vi "run.vi"() -> ()   [LabVIEW 2010, in "AnalysisRaps2.lvclass"]
uses:
  AnalysisRaps2.lvclass
  common/classes/ErrorController/ErrorController/ErrorController.lvclass
  common/classes/ImageCollection/ImageCollection/ImageCollection.lvclass
  AnalysisRaps2.lvclass/AnalysisRaps2.ctl
  common/classes/ErrorController/ErrorController/class_data.vi
panel:
  out "average":sgl[](graph) caption="graph r"
  in  "stop":bool
  out "graph r":sgl[][](graph)
  out "r0":sgl[](array[numeric])
  in  "r0 end point":i32=1
  in  "r0 start point":i32
  in  "# rolling average":i32=1 min=1
  in  "extra offset":dbl=10.0
  in  "show index":i32
  out "single graph":sgl[](graph)
  out "graph blue":sgl[][](graph)
  in  "# lines to skip":i32
  out "graph yellow":sgl[][](graph)
  in  "# subpatterns":i32=1 min=1
  out "progress slider":u8(slide) scale=0.0..100.0
  in  "channel: yellow":i32=1
  in  "channel: blue":i32
  out "error out":errorcluster
  in  "Path":path
  out "error handler":bool
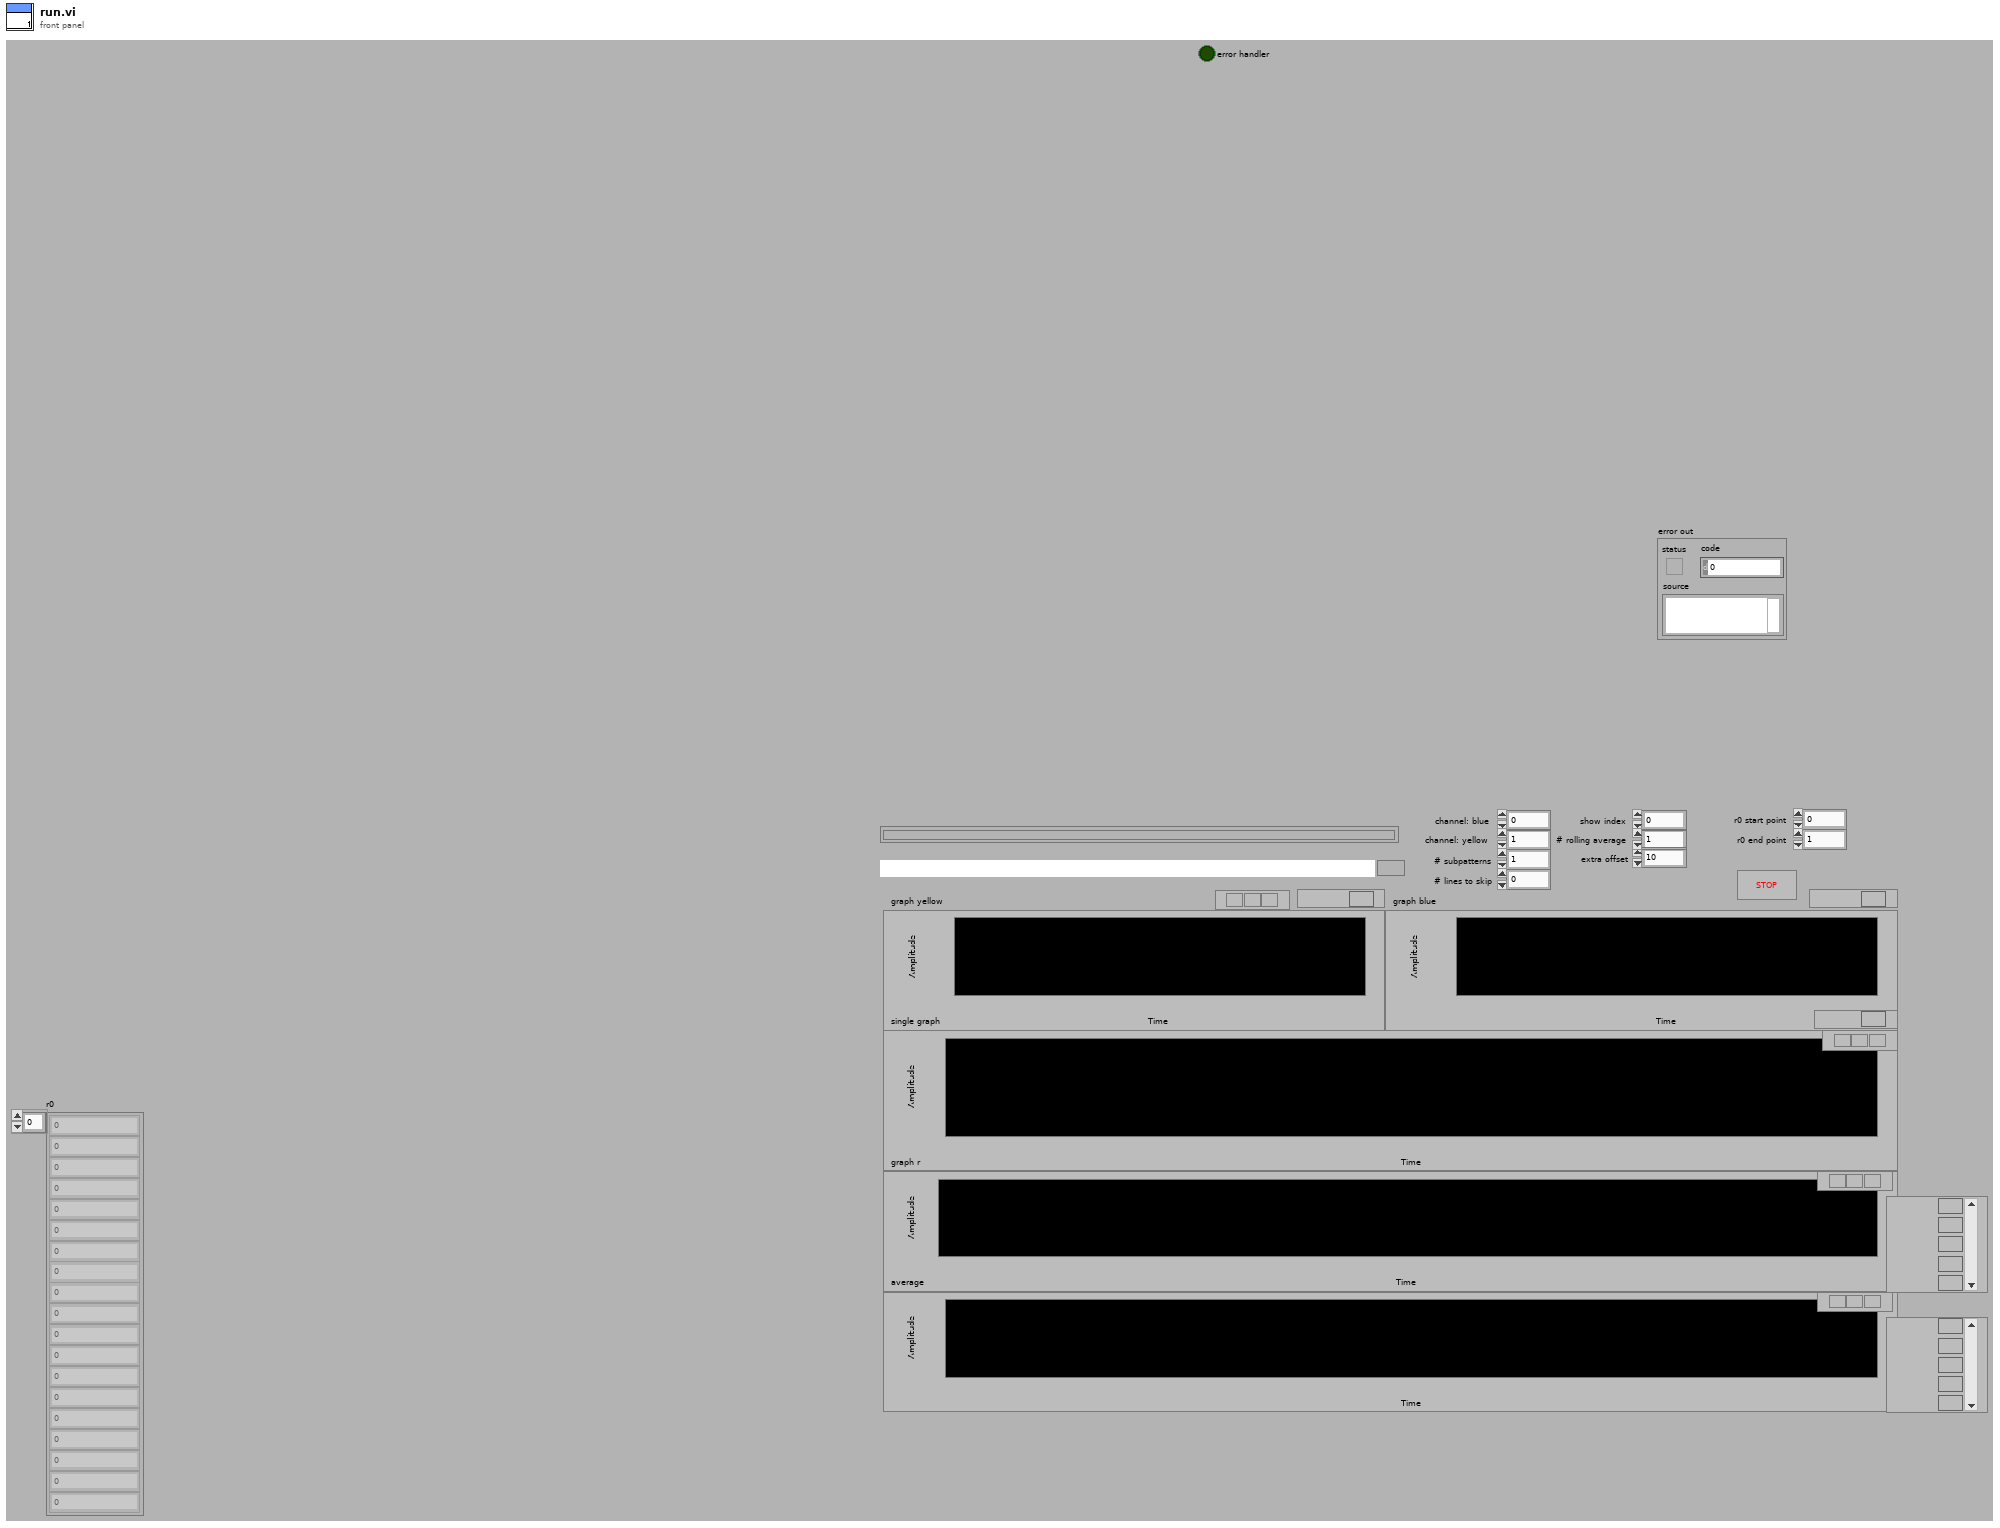
[diagram p1: front panel]
types:
  T1 = typedef "Image Type" = u32
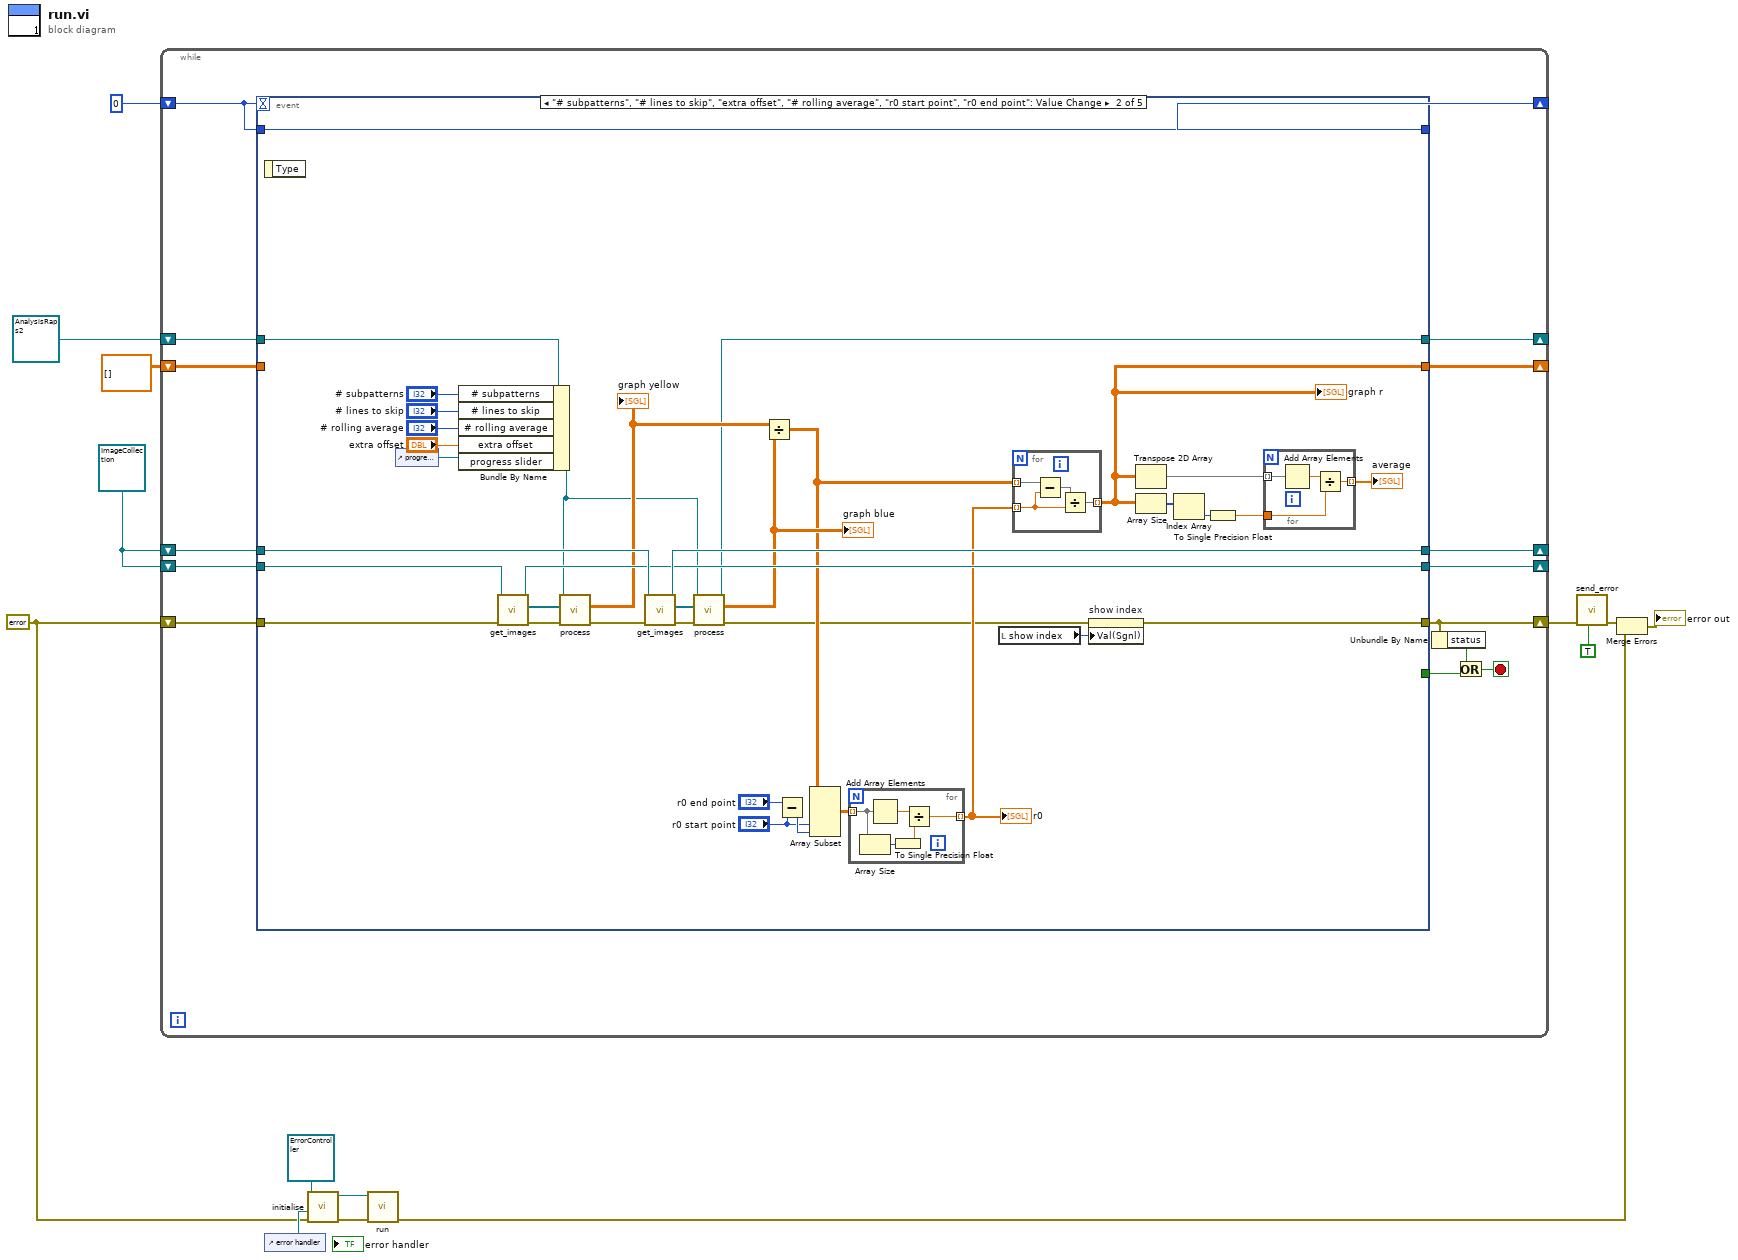
[diagram p0: block diagram]
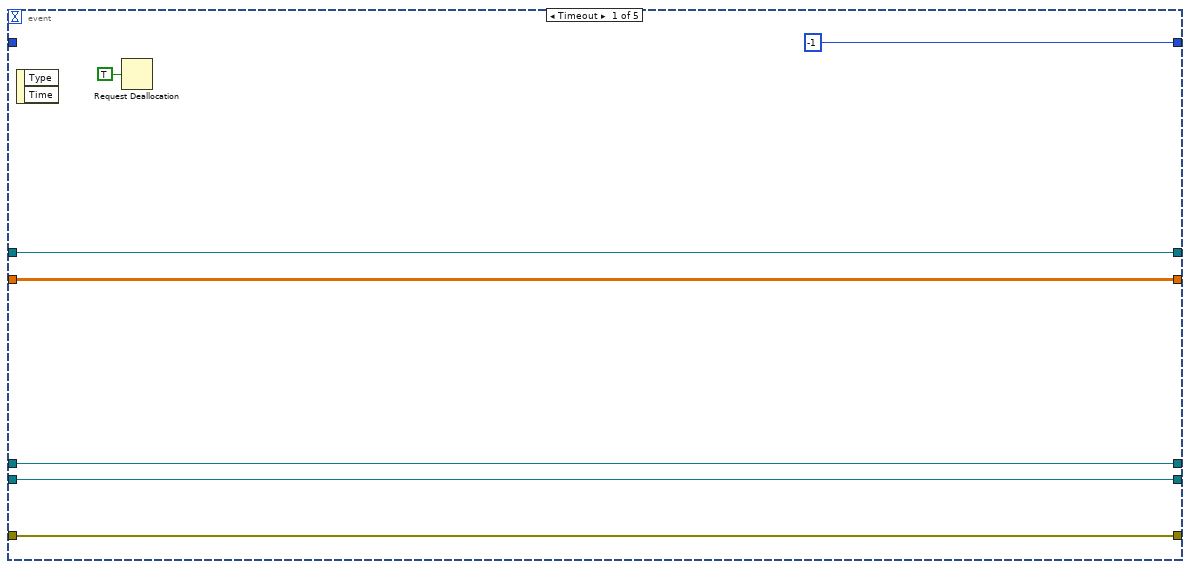
[diagram p2: hidden frame]
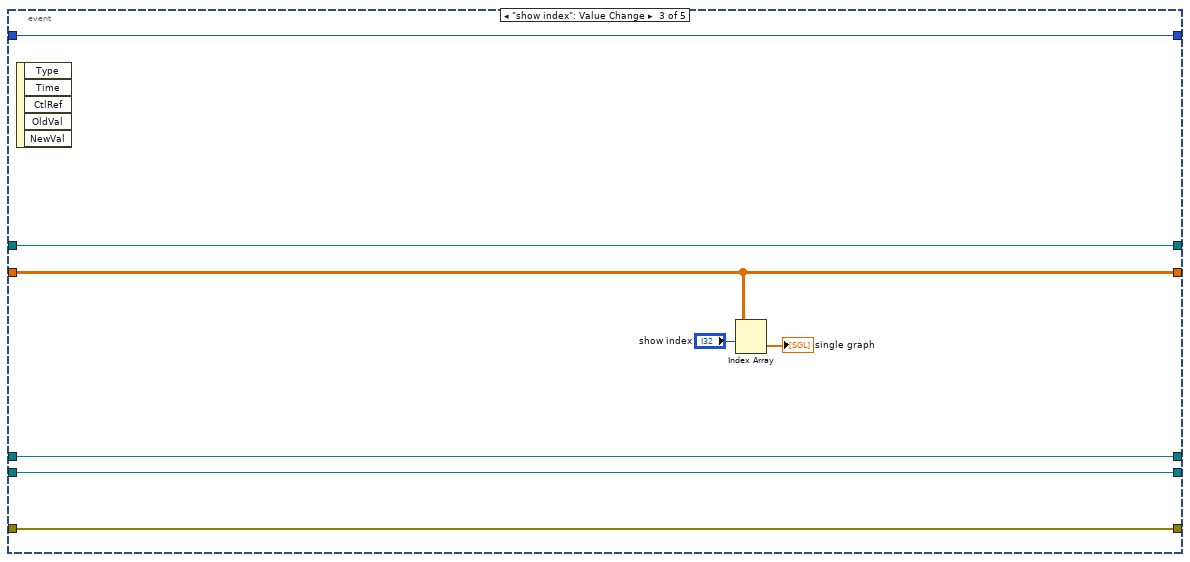
[diagram p3: hidden frame]
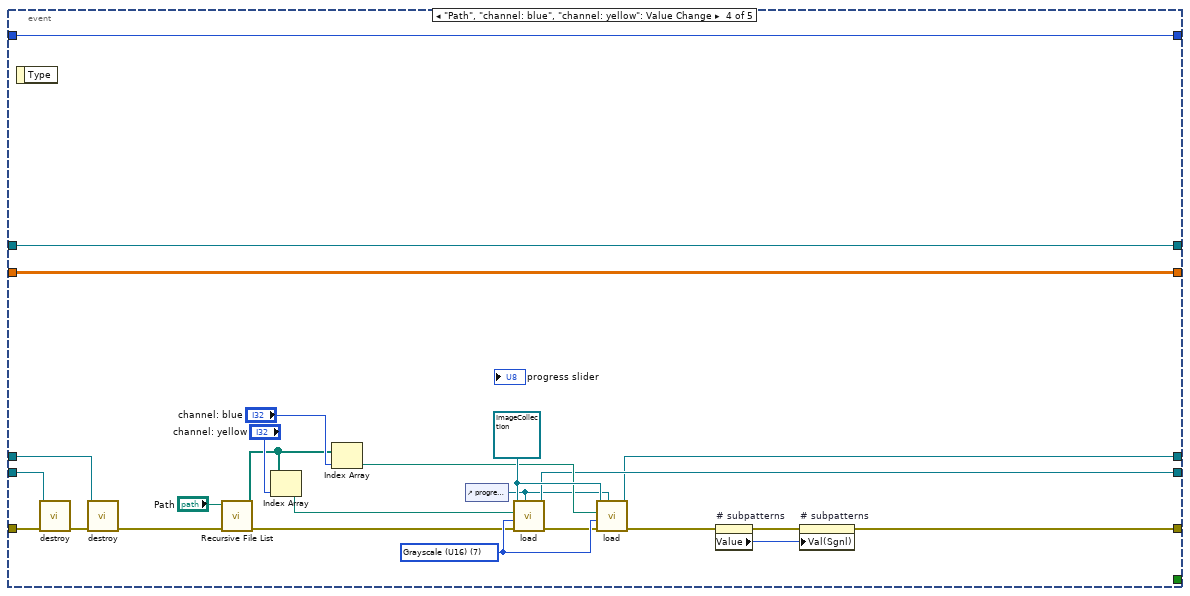
[diagram p4: hidden frame]
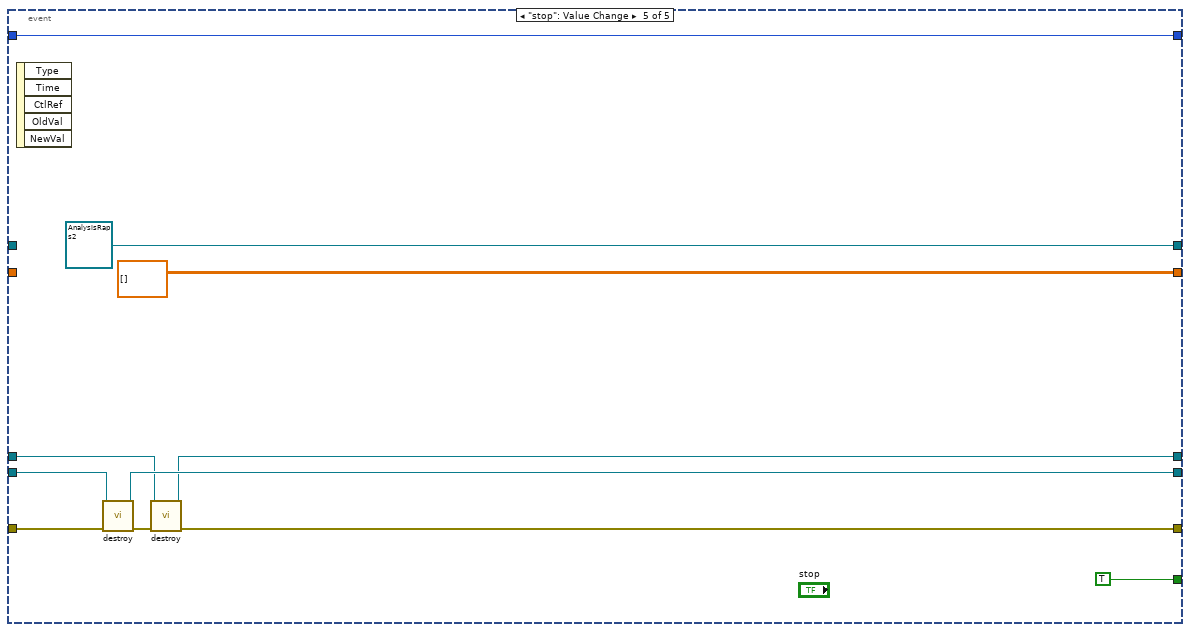
[diagram p5: hidden frame]
diagram:
  w1 = refnum<class "ImageCollection.lvclass"> refnum ("ImageCollection out")
  w9 = errorcluster {"status"=FALSE, "code"=0, "source"=""} ("error in (no error)")
  n1 = while {
    shift-right: [w29] -> _
    shift-left: 0 -> [w28]
    shift-right: [w18] -> w7
    shift-left: w9 -> [w27]
    shift-right: [w25] -> _
    shift-left: refnum<class "AnalysisRaps2.lvclass"> refnum ("AnalysisRaps2.lvclass") -> [w26]
    shift-right: [w22] -> _
    shift-left: w1 -> [w23]
    shift-right: [w21] -> _
    shift-left: w1 -> [w24]
    shift-right: [w20] -> _
    shift-left: sgl[][] [] -> [w19]
    stop <- w15 stop-if-true
    n2 = event shown="[1] \"# subpatterns\", \"# lines to skip\", \"extra offset\", \"# rolling average\", \"r0 start point\", \"r0 end point\": Value Change" {
      selector: _ -> [_ _ _ _ _]
      dyn-events: _ -> [_ _ _ _ _]
      timeout: w28 -> [_ _ _ _ _]
      tunnel: [-1 w72 w93 w118 w129] -> w29
      tunnel: w28 -> [_ w72 w93 w118 w129]
      tunnel: w27 -> [w34 w47 w92 w103 w126]
      tunnel: [w34 w49 w92 w97 w125] -> w18
      tunnel: w26 -> [w33 w60 w91 w117 _]
      tunnel: [w33 w61 w91 w117 refnum<class "AnalysisRaps2.lvclass"> refnum ("AnalysisRaps2.lvclass")] -> w25
      tunnel: [w32 w70 w90 w108 w121] -> w22
      tunnel: w24 -> [w31 w68 w89 w105 w124]
      tunnel: w23 -> [w32 w69 w90 w101 w122]
      tunnel: [w31 w66 w89 w109 w123] -> w21
      tunnel: [w30 w37 w87 w96 sgl[][] []] -> w20
      tunnel: w19 -> [w30 _ w87 w96 _]
      tunnel: [_ _ _ _ TRUE] -> w16
      event Timeout {
        n3 = event-data() -> ()  [unwired: 1 in, 2 out]
        n4 = Request Deallocation(TRUE ("flag")) -> ()
      }
      event "# subpatterns", "# lines to skip", "extra offset", "# rolling average", "r0 start point", "r0 end point": Value Change {
        n5 = event-data() -> ()  [unwired: 1 in, 1 out]
        n6 = control-ref of="progress slider"() -> (w43:refnum<vi>)
        n7 = Bundle By Name(cluster=w60, "# subpatterns"="# subpatterns", "# lines to skip"="# lines to skip", "# rolling average"="# rolling average", "extra offset"="extra offset", "progress slider"=w43) -> (w46:refnum<class "AnalysisRaps2.lvclass">)
        n8 = call-dynamic "get_images.vi"("error in (no error)"=w47, "ImageCollection.lvclass in"=w68) -> ("error out"=w67:errorcluster, "images"=w63:refnum<class "Image.lvclass">[], "ImageCollection.lvclass out"=w66:refnum<class "ImageCollection.lvclass">)  [unwired: 7 in]
        n9 = call "process.vi"("error in"=w67, "images"=w63, "AnalysisRaps2.lvclass 2"=w46) -> ("error out"=w45:errorcluster, "Array"=w65:sgl[][])  [unwired: 6 in, 1 out]
        "graph yellow" <- w65
        n10 = call-dynamic "get_images.vi"("error in (no error)"=w45, "ImageCollection.lvclass in"=w69) -> ("error out"=w71:errorcluster, "images"=w62:refnum<class "Image.lvclass">[], "ImageCollection.lvclass out"=w70:refnum<class "ImageCollection.lvclass">)  [unwired: 7 in]
        n11 = call "process.vi"("error in"=w71, "images"=w62, "AnalysisRaps2.lvclass 2"=w46) -> ("error out"=w44:errorcluster, "Array"=w64:sgl[][], "AnalysisRaps2.lvclass"=w61:refnum<class "AnalysisRaps2.lvclass">)  [unwired: 6 in]
        "graph blue" <- w64
        n12 = Divide(x=w65, y=w64) -> (x/y=w50:sgl[][])
        n13 = Subtract(x="r0 end point", y="r0 start point") -> (x-y=w54:i32)
        n14 = Array Subset(array=w50, index (col)="r0 start point", length (col)=w54) -> (w55:sgl[][])  [unwired: 2 in]
        n15 = for {
          tunnel: w55 -> [w84] mode=indexing
          tunnel: [w81] -> w51 mode=indexing
          n16 = Array Size(array=w84) -> (size(s)=w83:i32)
          n17 = Add Array Elements(numeric array=w84) -> (sum=w85:sgl)
          n18 = To Single Precision Float(number=w83) -> (single precision float=w82:sgl)
          n19 = Divide(x=w85, y=w82) -> (x/y=w81:sgl)
        }
        "r0" <- w51
        n20 = local read "show index"() -> (w48:i32)
        n21 = for {
          tunnel: w50 -> [w80] mode=indexing
          tunnel: w51 -> [w79] mode=indexing
          tunnel: [w77] -> w37 mode=indexing
          n22 = Subtract(x=w80, y=w79) -> (x-y=w78:sgl[])
          n23 = Divide(x=w78, y=w79) -> (x/y=w77:sgl[])
        }
        "graph r" <- w37
        n24 = property on="show index" class="DigNum (strict)"(error in=w44, "Val(Sgnl)"=w48) -> (error out=w49:errorcluster)  [unwired: 1 in, 1 out]
        n25 = Transpose 2D Array(2D array=w37) -> (transposed array=w41:sgl[][])
        n26 = Array Size(array=w37) -> (size(s)=w40:i32[])
        n27 = Index Array(array=w40) -> (element=w39:i32)  [unwired: 1 in]
        n28 = To Single Precision Float(number=w39) -> (single precision float=w38:sgl)
        n29 = for {
          tunnel: w41 -> [w74] mode=indexing
          tunnel: [w75] -> w42 mode=indexing
          tunnel: w38 -> [w73]
          n30 = Add Array Elements(numeric array=w74) -> (sum=w76:sgl)
          n31 = Divide(x=w76, y=w73) -> (x/y=w75:sgl)
        }
        "average" <- w42
      }
      event "show index": Value Change {
        n32 = event-data() -> ()  [unwired: 1 in, 5 out]
        n33 = Index Array(array=w87, index (row)="show index") -> (element=→"single graph":sgl[])  [unwired: 1 in]
      }
      event "Path", "channel: blue", "channel: yellow": Value Change {
        w106 = T1 7 items=["Grayscale (U8)", "Grayscale (I16)", "Grayscale (SGL)", "Complex (CSG)", "RGB (U32)", "HSL (U32)", "RGB (U64)", "Grayscale (U16)"] ("Image Type")
        w112 = refnum<class "ImageCollection.lvclass"> refnum ("ImageCollection in")
        n34 = event-data() -> ()  [unwired: 1 in, 1 out]
        n35 = call-dynamic "destroy.vi"("error in (no error)"=w103, "ImageCollection in"=w105) -> ("error out"=w104:errorcluster)  [unwired: 8 in, 1 out]
        n36 = call-dynamic "destroy.vi"("error in (no error)"=w104, "ImageCollection in"=w101) -> ("error out"=w102:errorcluster)  [unwired: 8 in, 1 out]
        n37 = call <vilib>:"Recursive File List.vi"("error in (no error)"=w102, "Folder Path"="Path") -> ("error out"=w95:errorcluster, "All Files in Dir"=w113:path[])  [unwired: 5 in, 3 out]
        n38 = Index Array(array=w113, index="channel: yellow") -> (element=w111:path)
        n39 = Index Array(array=w113, index="channel: blue") -> (element=w110:path)
        n40 = control-ref of="progress slider"() -> (w107:refnum<vi>)
        n41 = call "load.vi"("progress bar ref"=w107, "error in (no error)"=w95, "Image Type"=w106, "path in"=w111, "ImageCollection in"=w112) -> ("error out"=w94:errorcluster, "ImageCollection out"=w109:refnum<class "ImageCollection.lvclass">)  [unwired: 2 in, 3 out]
        n42 = call "load.vi"("progress bar ref"=w107, "error in (no error)"=w94, "Image Type"=w106, "path in"=w110, "ImageCollection in"=w112) -> ("error out"=w98:errorcluster, "ImageCollection out"=w108:refnum<class "ImageCollection.lvclass">)  [unwired: 2 in, 3 out]
        n43 = property on="# subpatterns" class="DigNum (strict)"(error in=w98) -> (error out=w99:errorcluster, "Value"=w100:i32)  [unwired: 1 in, 1 out]
        n44 = property on="# subpatterns" class="DigNum (strict)"(error in=w99, "Val(Sgnl)"=w100) -> (error out=w97:errorcluster)  [unwired: 1 in, 1 out]
      }
      event "stop": Value Change {
        n45 = event-data() -> ()  [unwired: 1 in, 5 out]
        n46 = call-dynamic "destroy.vi"("error in (no error)"=w126, "ImageCollection in"=w124) -> ("error out"=w127:errorcluster, "ImageCollection out"=w123:refnum<class "ImageCollection.lvclass">)  [unwired: 8 in]
        n47 = call-dynamic "destroy.vi"("error in (no error)"=w127, "ImageCollection in"=w122) -> ("error out"=w125:errorcluster, "ImageCollection out"=w121:refnum<class "ImageCollection.lvclass">)  [unwired: 8 in]
      }
    }
    n48 = Unbundle By Name(w18) -> ("status"=w17:bool)
    n49 = Or(x=w17, y=w16) -> (x .or. y?=w15:bool)
  }
  n50 = control-ref of="error handler"() -> (w12:refnum<vi>)
  n51 = call-dynamic "initialise.vi"("error in (no error)"=w9, "error boolean"=w12, "ErrorController in"=refnum<class "ErrorController.lvclass"> refnum ("ErrorController.lvclass")) -> ("error out"=w13:errorcluster, "ErrorController out"=w14:refnum<class "ErrorController.lvclass">)  [unwired: 7 in]
  n52 = call "run.vi"("error in (no error)"=w13, "ErrorController in"=w14) -> ("error out"=w4:errorcluster)  [unwired: 8 in, 1 out]
  n53 = call "send_error.vi"("last error? (F)"=TRUE, "error in (no error)"=w7) -> ("error out"=w5:errorcluster)  [unwired: 9 in]
  n54 = Merge Errors(w5, w4) -> (→"error out":errorcluster)
